vi "Probe Hostname.vi"(11 "Network Address out":refnum<class "Hostname Network Address.lvclass">) -> (2 "addr":string, 3 "Boolean":bool)   [LabVIEW 2020, in "NI_WFCN.lvlib" / "Hostname Network Address.lvclass"]
doc: "Prints the specific type of a Generic Network Address, and its string representation."
uses:
  <vilib>/net/WFCN/Addressing/Hostname Network Address/Hostname Network Address.lvclass
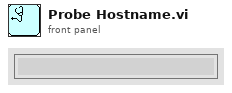
[diagram p1: front panel]
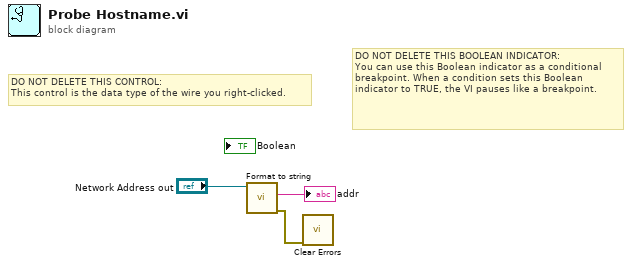
[diagram p0: block diagram]
diagram:
  # "DO NOT DELETE THIS BOOLEAN INDICATOR: \nYou can use this Boolean indicator as a conditional breakpoint. When a condition sets this Boolean indicator to TRUE, the VI pauses like a breakpoint."
  # "DO NOT DELETE THIS CONTROL: \nThis control is the data type of the wire you right-clicked."
  n1 = call-dynamic "Format to string.vi"("address"="Network Address out") -> ("error out"=w1:errorcluster, "String"=→"addr":string)  [unwired: 8 in, 1 out]
  n2 = call <vilib>:"Clear Errors.vi"("error in (no error)"=w1) -> ()  [unwired: 5 in, 2 out]
